vi "Write Config v1.1.vi"(8 "error in":errorcluster, 10 "All Para":cluster{"Auto Para":T1, "General Para 2":T2}={"Auto Para"={"Agitator Delays"=[250, 600], "TF Delays"=[400, 800, 2, 5000], "Insertion Delays"=[100, 400], "Cutting Delays"=[150, 250, 50], "PF Delays"=[320, 8000], "Measur. Delays"=[200.0, 188.9, 1.0], "Reject Delays"=[500], "BF Delays"=[1000, 1000], "P&P Delays"=[1000]}, "General Para 2"={"Max. Cons."=5.0, "Offset 1"=0.0, "Offset 2"=0.0, "Offset 3"=0.0, "Offset 4"=-0.6, "OutputPause"=500.0, "RejectPause"=500.0, "IndexTimeout"=0.0}} {"General Para 2"."Offset 4" format="%.2f"; "General Para 2"."Offset 3" format="%.2f"; "General Para 2"."Offset 2" format="%.2f"; "General Para 2"."Offset 1" format="%.2f"}, 11 "file path":path) -> (0 "error out":errorcluster, 3 "file path out":path)   [LabVIEW 2021]
doc: "v1.0:\n- Added 2WR bool"
uses:
  RT/Controls/Auto Delays.ctl
  Controls/General Para.ctl
  <vilib>/Utility/config.llb/Write Key (Double).vi
  <vilib>/Utility/config.llb/Write Key (String).vi
  <vilib>/Utility/config.llb/NI_LVConfig.lvlib
panel:
  in  "password":string="1234"
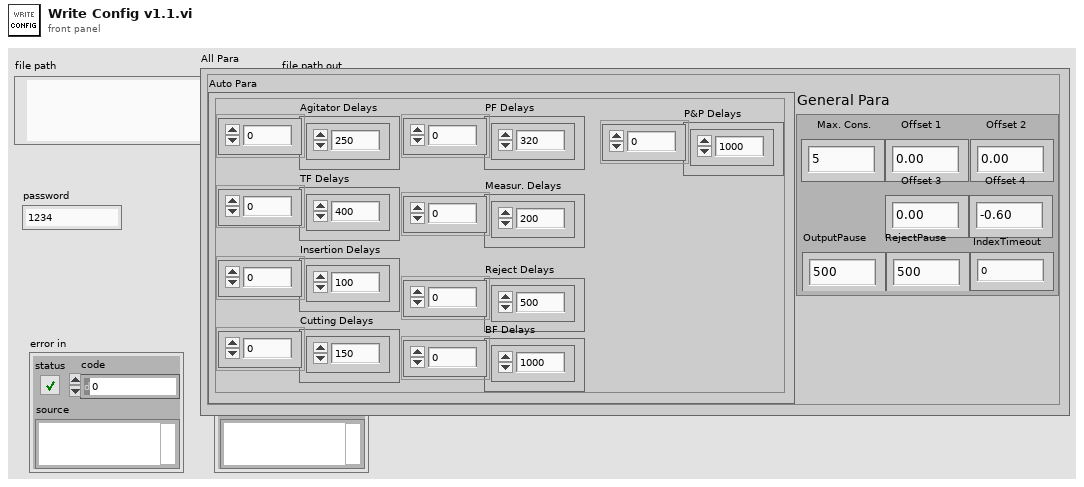
[diagram p1: front panel]
types:
  T1 = typedef "Auto Delays.ctl" = cluster{"Agitator Delays":u32[], "TF Delays":u32[], "Insertion Delays":u32[], "Cutting Delays":u32[], "PF Delays":u32[], "Measur. Delays":dbl[], "Reject Delays":u32[], "BF Delays":u32[], "P&P Delays":u32[]}
  T2 = typedef "General Para.ctl" = cluster{"Max. Cons.":dbl, "Offset 1":dbl, "Offset 2":dbl, "Offset 3":dbl, "Offset 4":dbl, "OutputPause":dbl, "RejectPause":dbl, "IndexTimeout":dbl}
  T3 = typedef "NI_LVConfig.lvlib/Config Data RefNum.ctl" = refnum<k1>
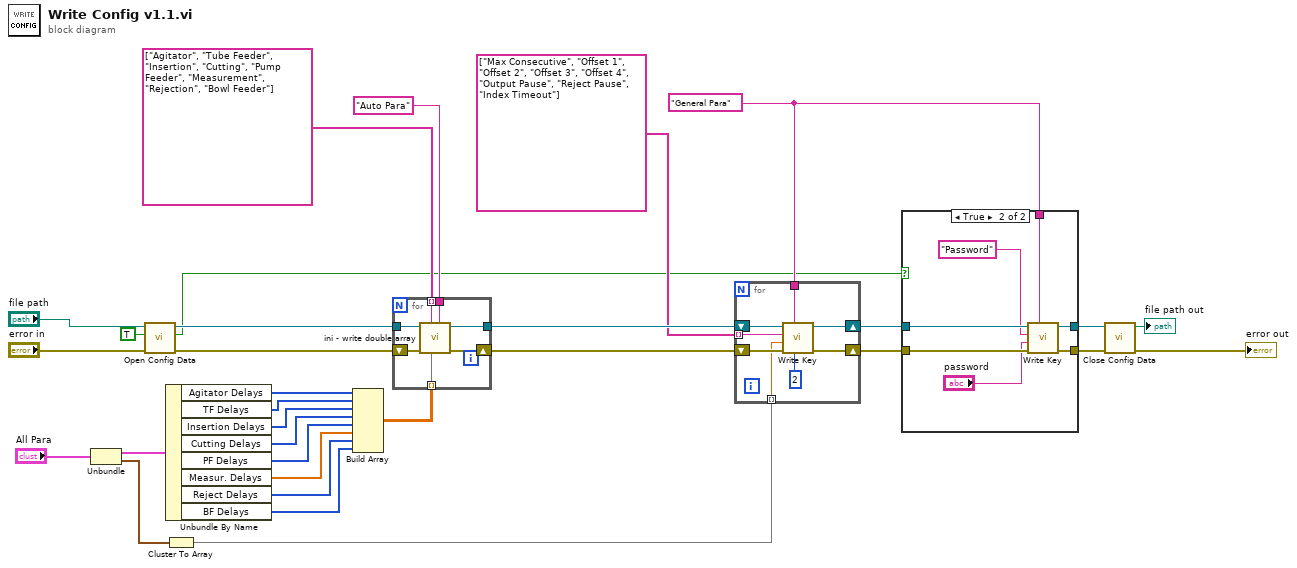
[diagram p0: block diagram]
diagram:
  w2 = "General Para" ("section")
  n1 = Unbundle("All Para") -> ("Auto Para"=w21:T1, "General Para 2"=w9:T2)
  n2 = call <vilib>:"Open Config Data.vi"("error in (no error)"="error in", "create file if necessary (T)"=TRUE, "configuration file path"="file path") -> ("error out"=w26:errorcluster, "file created?"=w1:bool, "refnum"=w27:T3)  [unwired: 6 in]
  n3 = Unbundle By Name(w21) -> ("Agitator Delays"=w20:u32[], "TF Delays"=w19:u32[], "Insertion Delays"=w18:u32[], "Cutting Delays"=w17:u32[], "PF Delays"=w16:u32[], "Measur. Delays"=w15:dbl[], "Reject Delays"=w14:u32[], "BF Delays"=w13:u32[])
  n4 = Cluster To Array(cluster=w9) -> (array=w8:dbl[])
  n5 = Build Array(w20, w19, w18, w17, w16, w15, w14, w13) -> (w12:dbl[][])
  n6 = for {
    tunnel: w27 -> [w38]
    tunnel: "Auto Para" ("section") -> [w34]
    tunnel: string[] ["Agitator", "Tube Feeder", "Insertion", "Cutting", "Pump Feeder", "Measurement", "Rejection", "Bowl Feeder"] -> [w33] mode=indexing
    tunnel: [w35] -> w11
    shift-right: [w36] -> w10
    shift-left: w26 -> [w37]
    tunnel: w12 -> [w32] mode=indexing
    n7 = call "ini - write double array.vi"("section"=w34, "double array"=w32, "key"=w33, "error in"=w37, "refnum in"=w38) -> ("error out"=w36:errorcluster, "refnum out"=w35:T3)  [unwired: 5 in]
  }
  n8 = for {
    tunnel: w2 -> [w44]
    shift-right: [w46] -> w4
    shift-left: w11 -> [w43]
    shift-right: [w45] -> w6
    shift-left: w10 -> [w42]
    tunnel: w8 -> [w41] mode=indexing
    tunnel: string[] ["Max Consecutive", "Offset 1", "Offset 2", "Offset 3", "Offset 4", "Output Pause", "Reject Pause", "Index Timeout"] -> [w40] mode=indexing
    n9 = call-poly <vilib>:"Write Key.vi"("precision (6)"=i16 2, "section"=w44, "error in (no error)"=w42, "value"=w41, "key"=w40, "refnum"=w43) -> ("error out"=w45:errorcluster, "refnum out"=w46:T3)  [unwired: 3 in, 1 out]
  }
  n10 = case shown="True" w1 {
    tunnel: w6 -> [w47 w55]
    tunnel: [w47 w54] -> w5
    tunnel: w4 -> [w48 w53]
    tunnel: [w48 w52] -> w3
    tunnel: w2 -> [_ w51]
    frame False {
    }
    frame True {
      n11 = call-poly <vilib>:"Write Key.vi"("section"=w51, "error in (no error)"=w55, "value"="password", "key"="Password", "refnum"=w53) -> ("error out"=w54:errorcluster, "refnum out"=w52:T3)  [unwired: 4 in, 1 out]
    }
  }
  n12 = call <vilib>:"Close Config Data.vi"("error in (no error)"=w5, "refnum"=w3) -> ("error out"=→"error out":errorcluster, "file path"=→"file path out":path)  [unwired: 8 in]
